vi "PXI-Pause DAQ.vi"() -> ()   [LabVIEW 2015]
uses:
  DAQ Engine VIs/PXI Globals.vi
panel:
  in  "Pause":bool
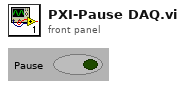
[diagram p1: front panel]
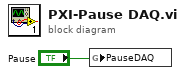
[diagram p0: block diagram]
diagram:
  n1 = global write "PXI Globals.vi" "PauseDAQ"("Pause") -> ()
